vi "Relativity.vi"() -> ()   [LabVIEW 2022 SP3]
panel:
  out "Relativistic Momentum (kgm/s)":dbl
  out "Relativistic Energy (J)":dbl
  out "Relativistic Mass (kg)":dbl
  in  "Rest mass (kg)":dbl
  in  "Velocity (m/s)":dbl
  # "Relativity:\nFor an object moving near the speed of light,\ncompared to the observer, the mass, energy, \nand momentum deviate from classical derivation.\nEnter the speed of an object, and its mass when \nat rest to see its relativistic mass, energy, and \nmomentum."
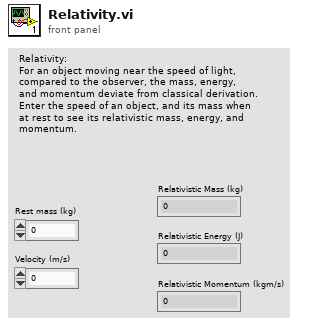
[diagram p1: front panel]
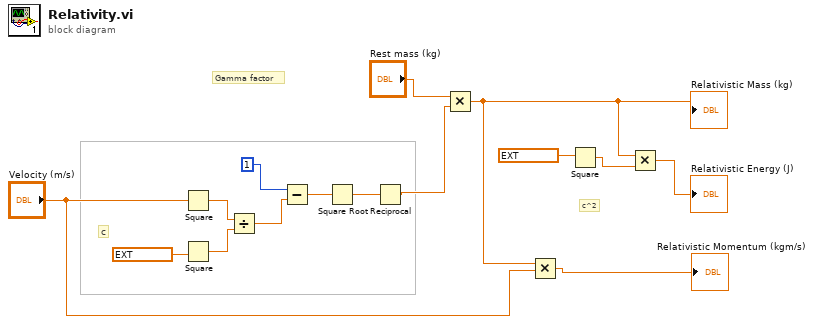
[diagram p0: block diagram]
diagram:
  # "c^2"
  # "c"
  # "Gamma factor"
  n1 = Square(x="Velocity (m/s)") -> (x^2=w14:dbl)
  n2 = Square(x=ext 299792458.0 ("Numeric")) -> (x^2=w13:ext)
  n3 = Divide(x=w14, y=w13) -> (x/y=w11:ext)
  n4 = Subtract(x=1, y=w11) -> (x-y=w10:ext)
  n5 = Square Root(x=w10) -> (sqrt(x)=w9:ext)
  n6 = Reciprocal(x=w9) -> (1/x=w8:ext)
  n7 = Multiply(x="Rest mass (kg)", y=w8) -> (x*y=w2:ext)
  "Relativistic Mass (kg)" <- w2
  n8 = Multiply(x=w2, y="Velocity (m/s)") -> (x*y=→"Relativistic Momentum (kgm/s)":ext)
  n9 = Square(x=ext 299792458.0 ("Numeric")) -> (x^2=w5:ext)
  n10 = Multiply(x=w2, y=w5) -> (x*y=→"Relativistic Energy (J)":ext)
